vi "Set_field_astrometry.vi"(0 "Cen x (pas)":i32=475000, 1 "effective rotation (°)":dbl step=5.0, 2 "scale (\"/pas)":dbl=0.00644, 3 "NaxisMax":i32=500000, 5 "Cen y (pas)":i32=475000, 7 "Use Center?":bool, 9 "Ref x (pas)":dbl=475000.0, 11 "Ref y (pas)":dbl=475000.0, 12 "RA (HH:MM:SS.S)":dbl format="%<%H:%M:%S%1u>t", 13 "DEC(DD:MM:SS)":dbl format="%<%H:%M:%S>t", 14 "Inversion Cluster":T1) -> (6 "Field Astrometry":T2={"NAXIS"=[53.666666666666664, 53.666666666666664], "CD"=[[0.016666666666666666, 0.0], [0.0, 0.016666666666666666]], "CDELT"=[1.0, 1.0], "CRPIX"=[1.0, 1.0], "CTYPE"=["RA---TAN", "DEC--TAN"], "CRVAL"=[0.0, 0.0], "LONGPOLE"=180.0, "LATPOLE"=90.0, "PV2"=[0.0, 0.0]}, 10 "Table Astrometry":T2={"NAXIS"=[500000.0, 500000.0], "CD"=[[0.0, -0.0], [0.0, 0.0]], "CDELT"=[1.0, 1.0], "CRPIX"=[475001.0, 475001.0], "CTYPE"=["RA---TAN", "DEC--TAN"], "CRVAL"=[0.0, 0.0], "LONGPOLE"=180.0, "LATPOLE"=90.0, "PV2"=[0.0, 0.0]})   [LabVIEW 2019]
uses:
  <vilib>/Analysis/baseanly.llb/Real Determinant.vi
  <vilib>/Analysis/Matrix/Numeric/Conversions/Array To Matrix - RA2.vi
  <vilib>/Analysis/Matrix/NI_Matrix.lvlib
  <vilib>/Analysis/NI_AALBase.lvlib
panel:
  out "Scale":dbl=1.788888888888889e-06
  out "scale (\"/px)":dbl
  # "ici, il s'agit d'une struture normale d'astrométrie, mais les pixels\nsont remplacés par des \"pas\" sur les tables de guidage et la \nrotation se fait à partir des pas correspondant au centre optique."
  # "y"
  # "DEC"
  # "x"
  # "RA"
  # "Position de référence"
  # "Valeurs synchronisées"
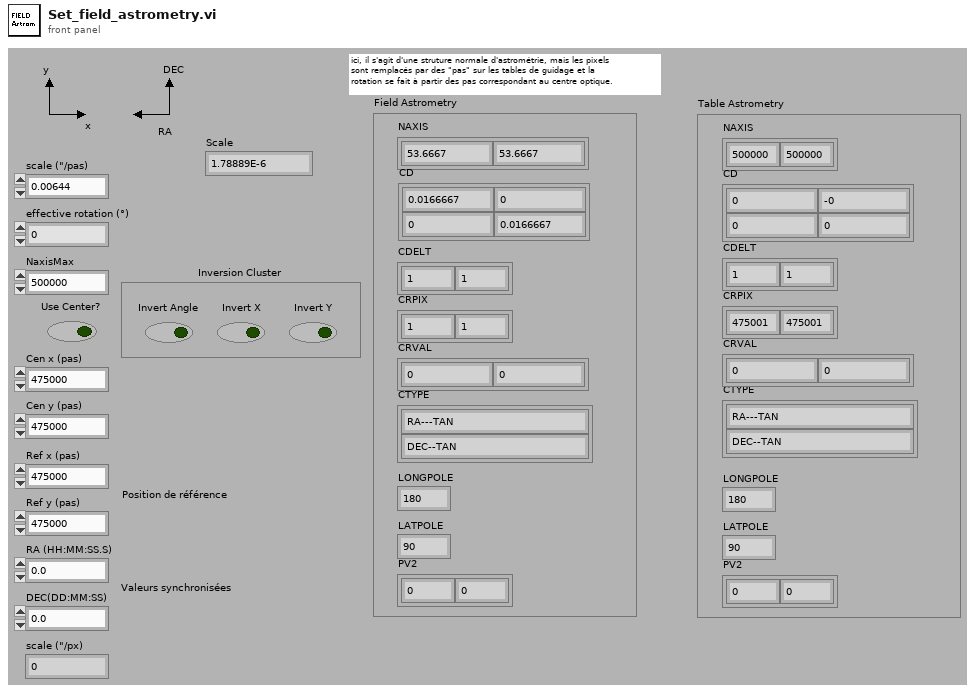
[diagram p1: front panel]
types:
  T1 = cluster{"Invert Angle":bool, "Invert X":bool, "Invert Y":bool}
  T2 = cluster{"NAXIS":dbl[], "CD":dbl[][], "CDELT":dbl[], "CRPIX":dbl[], "CTYPE":string[], "CRVAL":dbl[], "LONGPOLE":dbl, "LATPOLE":dbl, "PV2":dbl[]}
  T3 = typedef "NI_Matrix.lvlib/RealMatrix.ctl" = dbl[][]
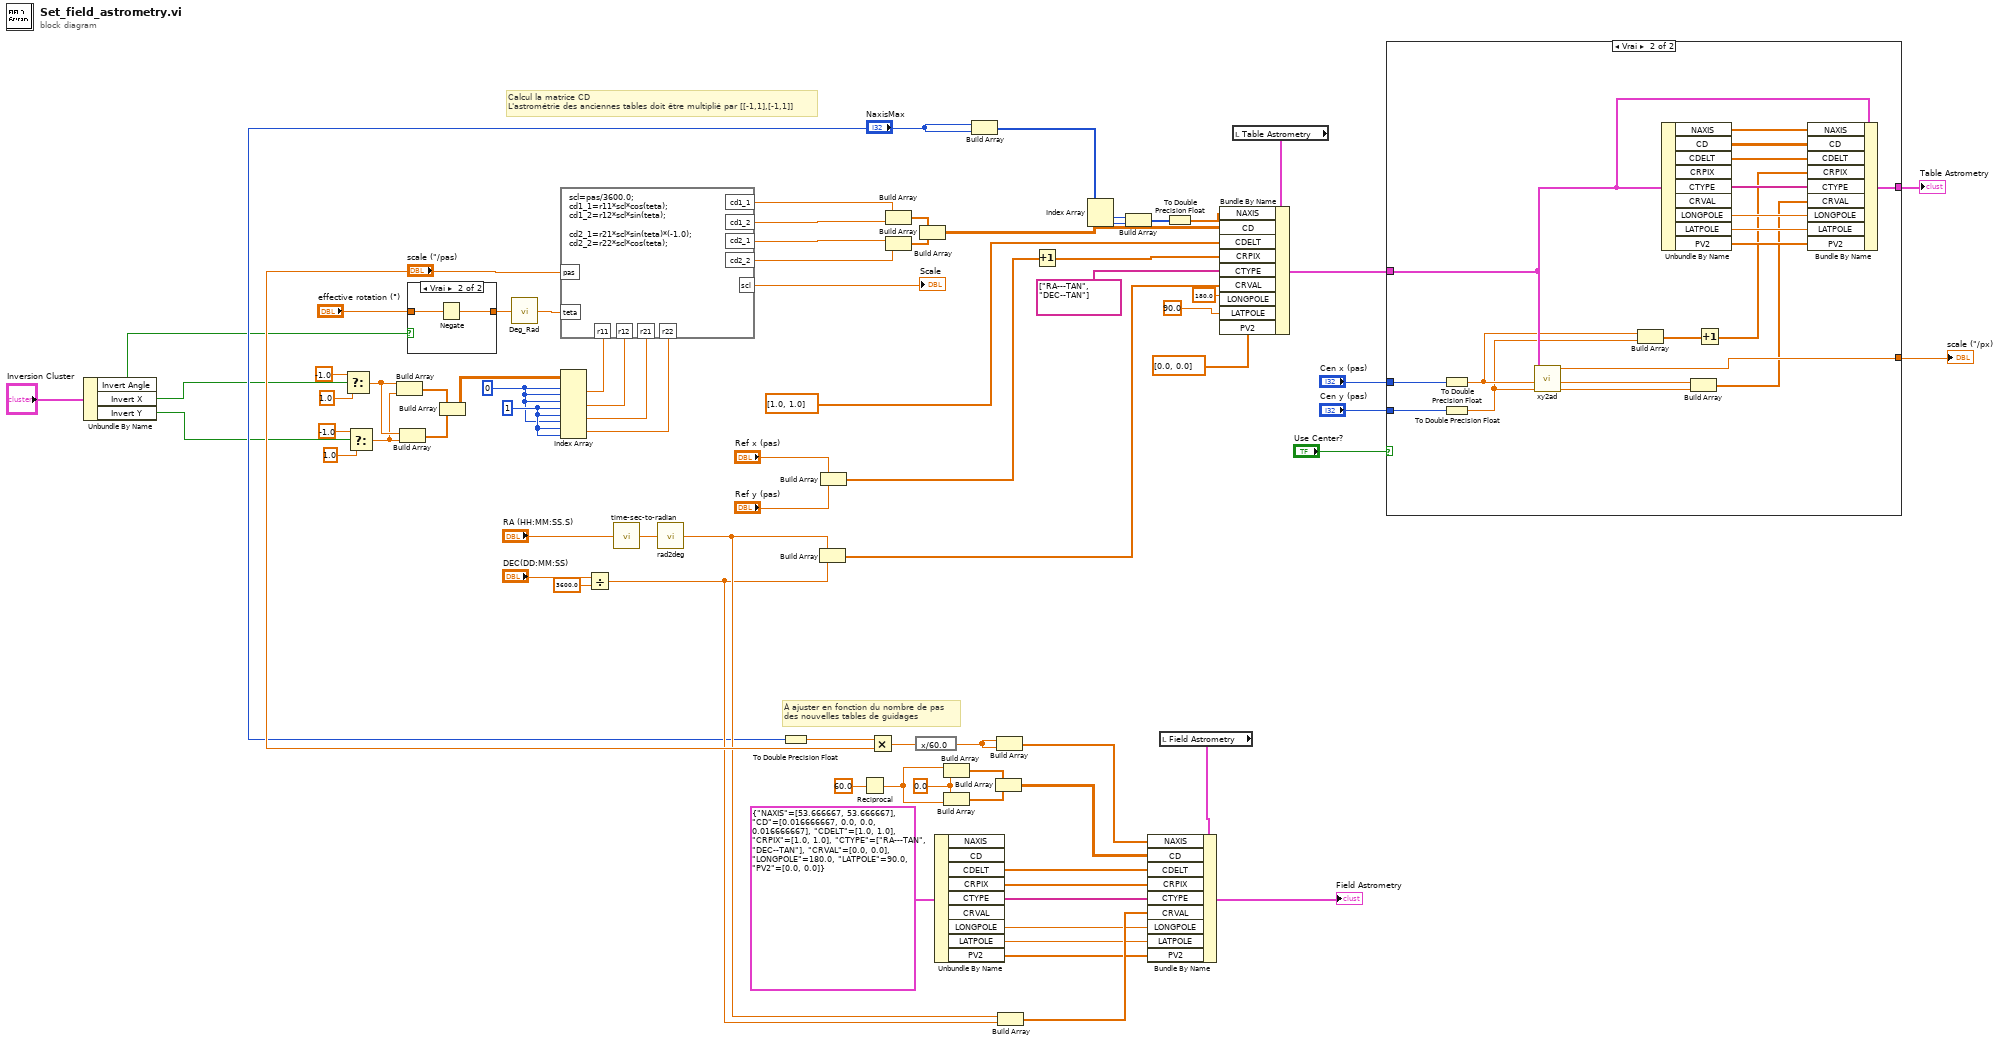
[diagram p0: block diagram]
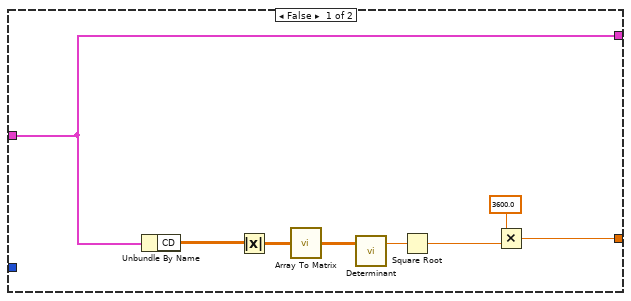
[diagram p3: hidden frame]
diagram:
  w21 = 1 ("disabled index (col)")
  w20 = 0 ("index (row)")
  w39 = 0.0 ("x")
  # "À ajuster en fonction du nombre de pas\ndes nouvelles tables de guidages"
  # "Calcul la matrice CD\nL'astrométrie des anciennes tables doit être multiplié par [[-1,1],[-1,1]]"
  n1 = Unbundle By Name("Inversion Cluster") -> ("Invert Angle"=w3:bool, "Invert X"=w5:bool, "Invert Y"=w4:bool)
  n2 = Select(t=-1.0, s=w5, f=1.0 ("t")) -> (s? t:f=w12:dbl)
  n3 = Select(t=-1.0, s=w4, f=1.0 ("t")) -> (s? t:f=w9:dbl)
  n4 = Build Array(w12, w9) -> (w7:dbl[])
  n5 = Build Array(w12, w9) -> (w8:dbl[])
  n6 = case shown="Vrai" w3 {
    tunnel: "effective rotation (°)" -> [w81 w83]
    tunnel: [w81 w82] -> w1
    frame False {
    }
    frame True {
      n7 = Negate(x=w83) -> (-x=w82:dbl)
    }
  }
  n8 = Build Array(w7, w8) -> (w15:dbl[][])
  n9 = call "Deg_Rad.vi"("Angle"=w1) -> ("RadRot"=w79:dbl)
  n10 = Index Array(array=w15, index (row) #1=w20, index (col) #1=w20, index (row) #2=w20, index (col) #2=w21, index (row) #3=w21, index (col) #3=w20, index (row) #4=w21, index (col) #4=w21) -> (element #1=w25:dbl, element #2=w24:dbl, element #3=w23:dbl, element #4=w22:dbl)
  n11 = formula code="scl=pas/3600.0;\ncd1_1=r11*scl*cos(teta);\ncd1_2=r12*scl*sin(teta);\n\ncd2_1=r21*scl*sin(teta)*(-1.0);\ncd2_2=r22*scl*cos(teta);"("teta"=w79, "pas"="scale (\"/pas)", "r11"=w25, "r12"=w24, "r21"=w23, "r22"=w22) -> ("cd1_1"=w16:dbl, "cd1_2"=w19:dbl, "cd2_1"=w18:dbl, "cd2_2"=w17:dbl, "scl"=→"Scale":dbl)
  n12 = Divide(x="DEC(DD:MM:SS)", y=3600.0) -> (x/y=w43:dbl)
  n13 = call "time-sec-to-radian.vi"("Numeric"="RA (HH:MM:SS.S)") -> ("radians"=w70:dbl)
  n14 = call "rad2deg.vi"("rad"=w70) -> ("deg"=w44:dbl)
  n15 = To Double Precision Float(number="NaxisMax") -> (double precision float=w27:dbl)
  n16 = Build Array(w44, w43) -> (w69:dbl[])
  n17 = Build Array("Ref x (pas)", "Ref y (pas)") -> (w72:dbl[])
  n18 = Reciprocal(x=60.0) -> (1/x=w38:dbl)
  n19 = Multiply(x=w27, y="scale (\"/pas)") -> (x*y=w42:dbl)
  n20 = Build Array(w16, w19) -> (w78:dbl[])
  n21 = Build Array(w18, w17) -> (w77:dbl[])
  n22 = expression code="x/60.0"(w42) -> (w41:dbl)
  n23 = Build Array(w78, w77) -> (w76:dbl[][])
  n24 = Unbundle By Name(T2 {"NAXIS"=[53.666667, 53.666667], "CD"=[[0.016666667, 0.0], [0.0, 0.016666667]], "CDELT"=[1.0, 1.0], "CRPIX"=[1.0, 1.0], "CTYPE"=["RA---TAN", "DEC--TAN"], "CRVAL"=[0.0, 0.0], "LONGPOLE"=180.0, "LATPOLE"=90.0, "PV2"=[0.0, 0.0]} ("Field_Astrom")) -> ("CDELT"=w55:dbl[], "CRPIX"=w54:dbl[], "CTYPE"=w53:string[], "LONGPOLE"=w51:dbl, "LATPOLE"=w50:dbl, "PV2"=w49:dbl[])  [unwired: 3 out]
  n25 = Build Array(w38, w39) -> (w37:dbl[])
  n26 = Build Array(w39, w38) -> (w36:dbl[])
  n27 = Build Array("NaxisMax", "NaxisMax") -> (w28:i32[])
  n28 = Build Array(w37, w36) -> (w35:dbl[][])
  n29 = Build Array(w41, w41) -> (w56:dbl[])
  n30 = Build Array(w44, w43) -> (w52:dbl[])
  n31 = Increment(x=w72) -> (x+1=w65:dbl[])
  n32 = Index Array(array=w28) -> (element #1=w34:i32, element #2=w33:i32)  [unwired: 2 in]
  n33 = Build Array(w34, w33) -> (w32:i32[])
  n34 = local read "Field Astrometry"() -> (w46:T2)
  n35 = Bundle By Name(cluster=w46, "NAXIS"=w56, "CD"=w35, "CDELT"=w55, "CRPIX"=w54, "CTYPE"=w53, "CRVAL"=w52, "LONGPOLE"=w51, "LATPOLE"=w50, "PV2"=w49) -> (→"Field Astrometry":T2)
  n36 = To Double Precision Float(number=w32) -> (double precision float=w64:dbl[])
  n37 = local read "Table Astrometry"() -> (w61:T2)
  n38 = Bundle By Name(cluster=w61, "NAXIS"=w64, "CD"=w76, "CDELT"=dbl[] [1.0, 1.0], "CRPIX"=w65, "CTYPE"=string[] ["RA---TAN", "DEC--TAN"], "CRVAL"=w69, "LONGPOLE"=180.0, "LATPOLE"=90.0, "PV2"=dbl[] [0.0, 0.0]) -> (w59:T2)
  n39 = case shown="Vrai" "Use Center?" {
    tunnel: [w84 w110] -> w80
    tunnel: w59 -> [w91 w97]
    tunnel: [w91 w96] -> w58
    tunnel: "Cen x (pas)" -> [_ w93]
    tunnel: "Cen y (pas)" -> [_ w92]
    frame False {
      n40 = Unbundle By Name(w91) -> ("CD"=w85:dbl[][])
      n41 = Absolute Value(x=w85) -> (abs(x)=w90:dbl[][])
      n42 = call-poly <vilib>:"Array To Matrix.vi"("Real 2D Array"=w90) -> ("Real Matrix"=w89:T3)
      n43 = call-poly <vilib>:"Determinant.vi"("Input Matrix"=w89) -> ("determinant"=w88:dbl)  [unwired: 1 in, 1 out]
      n44 = Square Root(x=w88) -> (sqrt(x)=w86:dbl)
      n45 = Multiply(x=3600.0, y=w86) -> (x*y=w84:dbl)
    }
    frame True {
      n46 = To Double Precision Float(number=w93) -> (double precision float=w95:dbl)
      n47 = To Double Precision Float(number=w92) -> (double precision float=w94:dbl)
      n48 = call "xy2ad.vi"("Y (px)"=w94, "X (px)"=w95, "Astrometry"=w97) -> ("DEC (°)"=w102:dbl, "RA (°)"=w101:dbl, "RA (HH:MM:SS.S)"=w110:dbl)  [unwired: 5 in, 1 out]
      n49 = Build Array(w95, w94) -> (w99:dbl[])
      n50 = Unbundle By Name(w97) -> ("NAXIS"=w103:dbl[], "CD"=w104:dbl[][], "CDELT"=w105:dbl[], "CTYPE"=w106:string[], "LONGPOLE"=w107:dbl, "LATPOLE"=w108:dbl, "PV2"=w109:dbl[])  [unwired: 2 out]
      n51 = Build Array(w101, w102) -> (w100:dbl[])
      n52 = Increment(x=w99) -> (x+1=w98:dbl[])
      n53 = Bundle By Name(cluster=w97, "NAXIS"=w103, "CD"=w104, "CDELT"=w105, "CRPIX"=w98, "CTYPE"=w106, "CRVAL"=w100, "LONGPOLE"=w107, "LATPOLE"=w108, "PV2"=w109) -> (w96:T2)
    }
  }
  "scale (\"/px)" <- w80
  "Table Astrometry" <- w58
